vi "MLLF_ClearTimeoutError.vi"(8 "error in (no error)":errorcluster) -> (0 "error out":errorcluster)   [LabVIEW 2018]
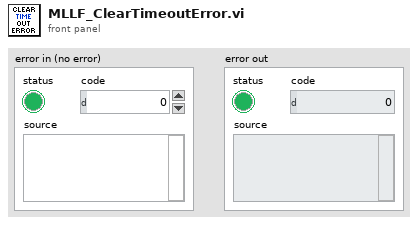
[diagram p1: front panel]
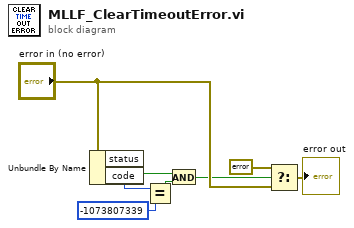
[diagram p0: block diagram]
diagram:
  n1 = Unbundle By Name("error in (no error)") -> ("status"=w6:bool, "code"=w3:i32)
  n2 = Equal?(x=w3, y=-1073807339) -> (x = y?=w5:bool)
  n3 = And(x=w6, y=w5) -> (x .and. y?=w7:bool)
  n4 = Select(t=errorcluster {"status"=FALSE, "code"=0, "source"=""} ("error IO"), s=w7, f="error in (no error)") -> (s? t:f=→"error out":errorcluster)
